vi "_088.vi"() -> ()   [LabVIEW 2024]
panel:
  out "o/p":dbl
  in  "index 3":i32
  in  "array 3":dbl[](array[numeric])
  out "o/p":dbl[](array[numeric])
  in  "index 2":i32
  in  "new element/\nsubarray 2":dbl
  in  "array 2":dbl[](array[numeric])
  out "o/p":dbl[](array[numeric])
  in  "new element/\nsubarray":dbl
  in  "index":i32
  in  "array":dbl[](array[numeric])
  out "o/p":dbl[](array[numeric])
  in  "dimension size":i32
  in  "element":dbl
  out "o/p":dbl
  # "Fundamentals :"
  # "17~>After running this VI,what is the value displayed in the o/p ?"
  # "Nrml Approach :"
  # "Initialize Array"
  # "Index Array"
  # "Insert in to  Array"
  # "Replace Array Subset"
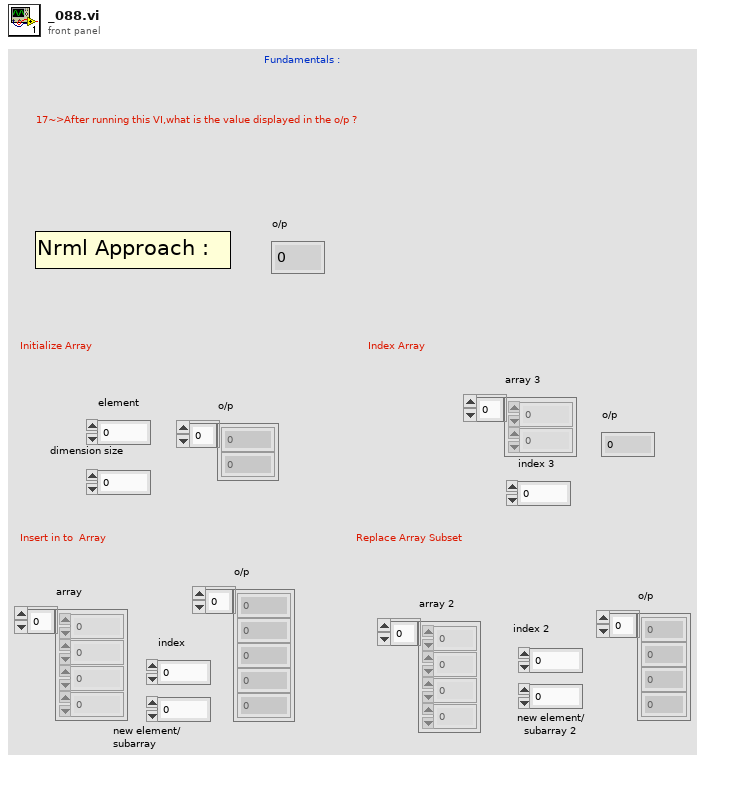
[diagram p1: front panel]
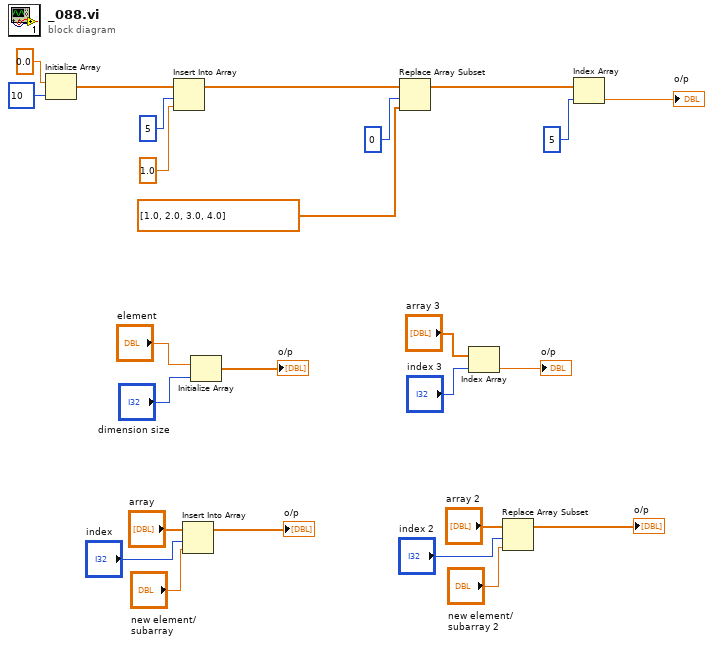
[diagram p0: block diagram]
diagram:
  n1 = Initialize Array "Initialize Array"(0.0 ("element"), 10 ("dimension size")) -> (w23:dbl[])
  n2 = Insert Into Array "Insert Into Array"(array=w23, index=5, new element=1.0 ("new element/subarray")) -> (w20:dbl[])
  n3 = Insert Into Array "Insert Into Array"(array="array", index="index", new element="new element/\nsubarray") -> (→"o/p":dbl[])
  n4 = Initialize Array "Initialize Array"("element", "dimension size") -> (→"o/p":dbl[])
  n5 = Replace Array Subset "Replace Array Subset"(array=w20, new element=dbl[] [1.0, 2.0, 3.0, 4.0] ("new element/subarray"), index=0) -> (w17:dbl[])
  n6 = Index Array "Index Array"(array="array 3", index="index 3") -> (element=→"o/p":dbl)
  n7 = Replace Array Subset "Replace Array Subset"(array="array 2", new element="new element/\nsubarray 2", index="index 2") -> (→"o/p":dbl[])
  n8 = Index Array "Index Array"(array=w17, index=5) -> (element=→"o/p":dbl)
